vi "PXIe-4139 Global Variable.vi"() -> ()   [LabVIEW 2023, in "PXIe-4139 Custom Device.lvlib"]
uses:
  PXIe-4139 Custom Device.lvlib
panel:
  in  "4139 page Disable GUID":string="98f307ac-acbe-4691-be32-87a99e80eb4e"
  in  "4139 page GUID":string="840c82ea-ae12-4c39-8450-d70da7ed9c17"
  in  "Continuous Read?":string="Continuous Read?"
  in  "Read Trigger":string="Read Trigger"
  in  "Channel #":string="Channel #"
  in  "Channel 0 Type":string="Channel 0 Type"
  in  "Channel 0 Sense":string="Channel 0 Sense"
  in  "Hardware Device Name":string="Hardware Device Name"
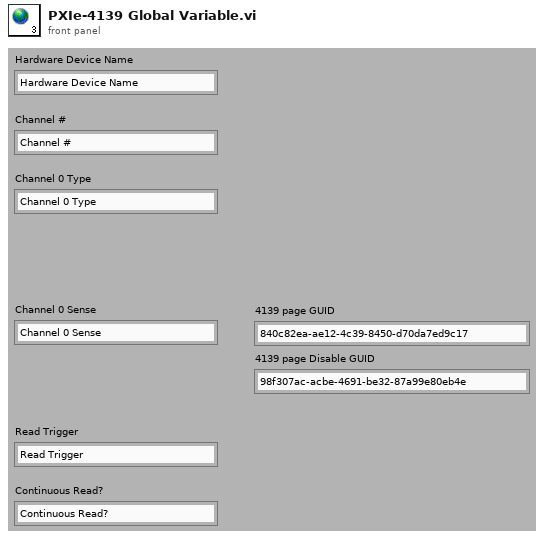
[diagram p1: front panel]
diagram:
